vi "Get Center of Sun.vi"(10 "Julian Century":dbl, 11 "Geometric Mean Anomaly":dbl) -> (3 "Sun Eq of Ctr":dbl)   [LabVIEW 2014, in "Solar Calculations.lvlib"]
uses:
  Solar Calculations.lvlib
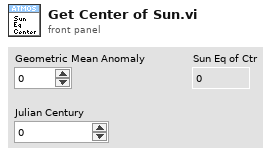
[diagram p1: front panel]
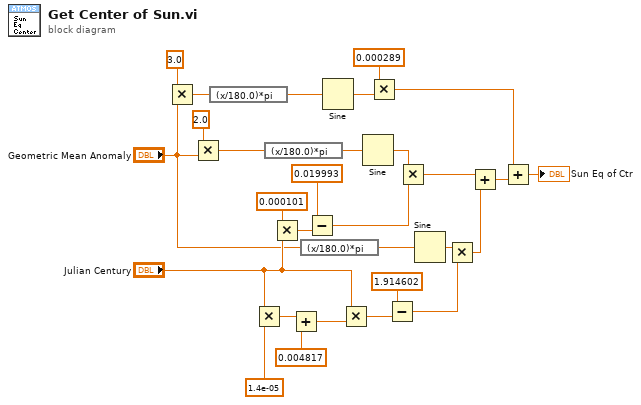
[diagram p0: block diagram]
diagram:
  n1 = Multiply(x=3.0, y="Geometric Mean Anomaly") -> (x*y=w6:dbl)
  n2 = Multiply(x=2.0, y="Geometric Mean Anomaly") -> (x*y=w4:dbl)
  n3 = expression code="(x/180.0)*pi" ("degrees to radians")(w6) -> (w5:dbl)
  n4 = Multiply(x="Julian Century", y=1.4e-05) -> (x*y=w9:dbl)
  n5 = expression code="(x/180.0)*pi" ("degrees to radians")(w4) -> (w3:dbl)
  n6 = Multiply(x=0.000101, y="Julian Century") -> (x*y=w18:dbl)
  n7 = Add(x=w9, y=0.004817) -> (x+y=w11:dbl)
  n8 = expression code="(x/180.0)*pi" ("degrees to radians")("Geometric Mean Anomaly") -> (w1:dbl)
  n9 = Subtract(x=0.019993, y=w18) -> (x-y=w20:dbl)
  n10 = Sine(x=w5) -> (sin(x)=w25:dbl)
  n11 = Multiply(x="Julian Century", y=w11) -> (x*y=w12:dbl)
  n12 = Sine(x=w3) -> (sin(x)=w21:dbl)
  n13 = Multiply(x=0.000289, y=w25) -> (x*y=w28:dbl)
  n14 = Subtract(x=1.914602, y=w12) -> (x-y=w14:dbl)
  n15 = Multiply(x=w21, y=w20) -> (x*y=w22:dbl)
  n16 = Sine(x=w1) -> (sin(x)=w15:dbl)
  n17 = Multiply(x=w15, y=w14) -> (x*y=w23:dbl)
  n18 = Add(x=w22, y=w23) -> (x+y=w27:dbl)
  n19 = Add(x=w28, y=w27) -> (x+y=→"Sun Eq of Ctr":dbl)
